vi "Acquire Data.vi"(7 "Total Buffer Size":i32, 8 "error in (no error)":errorcluster, 10 "Acquisition and Logging Configuration":T1={"Data Rate"=1, "Samples per Read"=0, "Number of Reads to Save"=0, "Data File Name"="", "TDMS Properties"=[], "Number of Channels"=4, "Channel Scale Array"=[0.0, 0.0, 0.0, 0.0], "Channel Names"=[], "Trigger - RMS Value"=0.0, "Trigger - Channel"=0, "Trigger - Time (Minute)"=0} {"Data Rate" items=["51.200 kS/s (NI 9234)"=1, "25.600 kS/s (NI 9234)"=2, "17.067 kS/s (NI 9234)"=3, "12.800 kS/s (NI 9234)"=4, "10.240 kS/s (NI 9234)"=5, "8.533 kS/s (NI 9234)"=6, "7.314 kS/s (NI 9234)"=7, "6.400 kS/s (NI 9234)"=8, "5.689 kS/s (NI 9234)"=9, "5.120 kS/s (NI 9234)"=10, "4.654 kS/s (NI 9234)"=11, "4.267 kS/s (NI 9234)"=12, "3.938 kS/s (NI 9234)"=13, "3.657 kS/s (NI 9234)"=14, "3.413 kS/s (NI 9234)"=15, "3.200 kS/s (NI 9234)"=16, "3.012 kS/s (NI 9234)"=17, "2.845 kS/s (NI 9234)"=18, "2.695 kS/s (NI 9234)"=19, "2.560 kS/s (NI 9234)"=20, "2.438 kS/s (NI 9234)"=21, "2.328 kS/s (NI 9234)"=22, "2.226 kS/s (NI 9234)"=23, "2.133 kS/s (NI 9234)"=24, "2.048 kS/s (NI 9234)"=25, "1.969 kS/s (NI 9234)"=26, "1.896 kS/s (NI 9234)"=27, "1.829 kS/s (NI 9234)"=28, "1.765 kS/s (NI 9234)"=29, "1.707 kS/s (NI 9234)"=30, "1.652 kS/s (NI 9234)"=31]}, 11 "FPGA VI Reference":T4) -> (0 "error out":errorcluster, 1 "Waveform Data":waveform(sgl)[](array[waveform]), 2 "dup Acquisition and Logging Configuration":T1={"Data Rate"=1, "Samples per Read"=0, "Number of Reads to Save"=0, "Data File Name"="", "TDMS Properties"=[], "Number of Channels"=4, "Channel Scale Array"=[0.0, 0.0, 0.0, 0.0], "Channel Names"=[], "Trigger - RMS Value"=0.0, "Trigger - Channel"=0, "Trigger - Time (Minute)"=0} {"Data Rate" items=["51.200 kS/s (NI 9234)"=1, "25.600 kS/s (NI 9234)"=2, "17.067 kS/s (NI 9234)"=3, "12.800 kS/s (NI 9234)"=4, "10.240 kS/s (NI 9234)"=5, "8.533 kS/s (NI 9234)"=6, "7.314 kS/s (NI 9234)"=7, "6.400 kS/s (NI 9234)"=8, "5.689 kS/s (NI 9234)"=9, "5.120 kS/s (NI 9234)"=10, "4.654 kS/s (NI 9234)"=11, "4.267 kS/s (NI 9234)"=12, "3.938 kS/s (NI 9234)"=13, "3.657 kS/s (NI 9234)"=14, "3.413 kS/s (NI 9234)"=15, "3.200 kS/s (NI 9234)"=16, "3.012 kS/s (NI 9234)"=17, "2.845 kS/s (NI 9234)"=18, "2.695 kS/s (NI 9234)"=19, "2.560 kS/s (NI 9234)"=20, "2.438 kS/s (NI 9234)"=21, "2.328 kS/s (NI 9234)"=22, "2.226 kS/s (NI 9234)"=23, "2.133 kS/s (NI 9234)"=24, "2.048 kS/s (NI 9234)"=25, "1.969 kS/s (NI 9234)"=26, "1.896 kS/s (NI 9234)"=27, "1.829 kS/s (NI 9234)"=28, "1.765 kS/s (NI 9234)"=29, "1.707 kS/s (NI 9234)"=30, "1.652 kS/s (NI 9234)"=31]})   [LabVIEW 2012]
doc: "Reads waveform data from the DMA FIFO."
uses:
  LabVIEW Data/FPGA Logging Test/controls/FPGA VI Reference.ctl
  LabVIEW Data/FPGA Logging Test/controls/Acquisition and Logging Configuration.ctl
  <vilib>/LabVIEW Targets/FPGA/cRIO/shared/nicrio_ModuleControls/nicrio_cRIO-9234_DataRatesRing2.ctl
  LabVIEW Data/FPGA Logging Test/controls/TDMS Properties.ctl
  LabVIEW Data/FPGA Logging Test/Globals/Global - Monitoring Variables.vi
  <vilib>/Utility/error.llb/Error Cluster From Error Code.vi
  <vilib>/rvi/errors/niLvFpgaAdjustHostInterfaceError.vi
  <vilib>/rvi/interface/nirviReadWriteControl/nirviReadWriteControl.xnode
  <vilib>/rvi/interface/nirviMethod/nirviMethod.xnode
  NiFpgaLv.dll
  <vilib>/rvi/interface/Simulation/niFpgaSimulationCallBeginRW.vi
  <vilib>/FPGAPlugInAG/Dynamic/niLvFpga_ReadFifo_Dynamic.vi
  <vilib>/rvi/errors/niLvFpgaMergeErrorWithErrorCode.vi
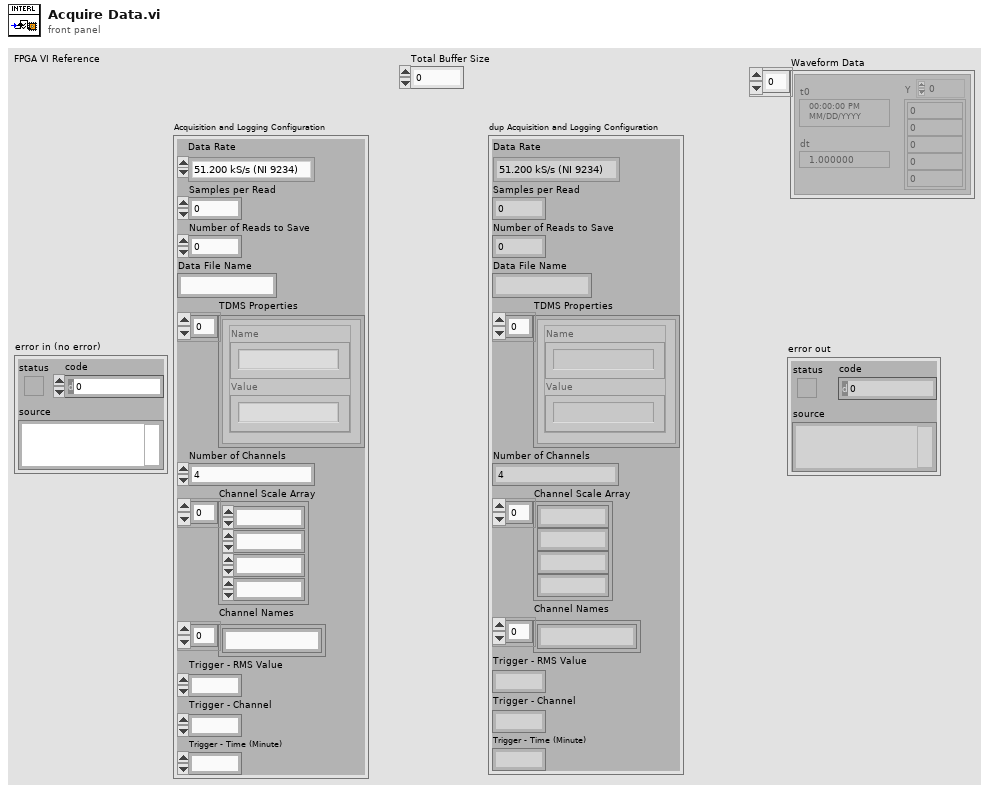
[diagram p1: front panel]
types:
  T1 = typedef "Acquisition and Logging Configuration.ctl" = cluster{"Data Rate":T2, "Samples per Read":i32, "Number of Reads to Save":i32, "Data File Name":string, "TDMS Properties":T3[], "Number of Channels":i32, "Channel Scale Array":fxp<+,24,12>[], "Channel Names":string[], "Trigger - RMS Value":dbl, "Trigger - Channel":i32, "Trigger - Time (Minute)":i32}
  T2 = typedef "nicrio_cRIO-9234_DataRatesRing2.ctl" = u8
  T3 = typedef "TDMS Properties.ctl" = cluster{"Name":string, "Value":string}
  T4 = typedef "FPGA VI Reference.ctl" = refnum<k20>
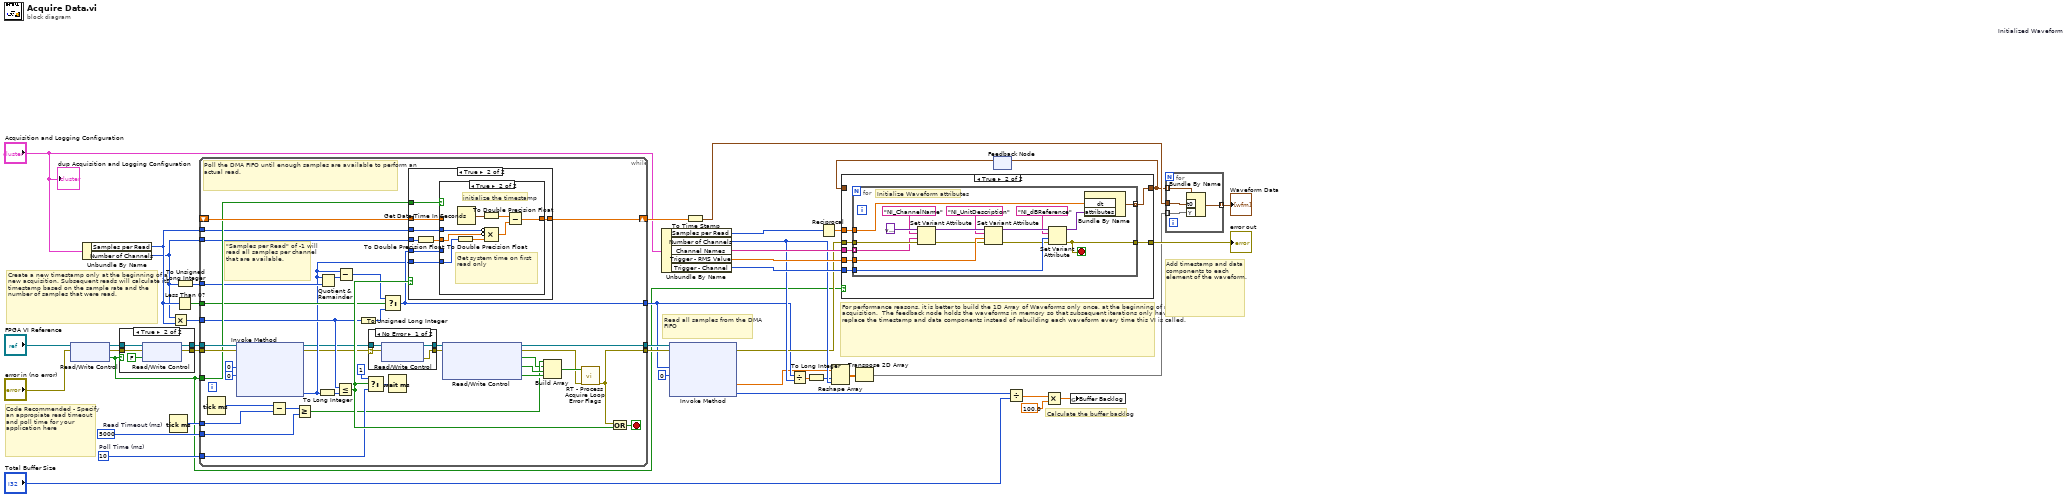
[diagram p0: block diagram]
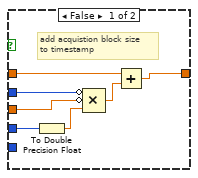
[diagram p5: hidden frame]
diagram:
  w13 = u32 10  # Poll Time (ms)
  w14 = u32 5000  # Read Timeout (ms)
  # "Calculate the buffer backlog"
  # "For performance reasons, it is better to build the 1D Array of Waveforms only once, at the beginning of an acquisition.  The feedback node holds the waveforms in memory so that subsequent iterations only have to replace the timestamp and data components instead of rebuilding each waveform every time this VI is called."
  # "Read all samples from the DMA FIFO"
  # "Code Recommended - Specify an appropiate read timeout and poll time for your application here"
  # "Create a new timestamp only at the beginning of a new acquisition. Subsequent reads will calculate its timestamp based on the sample rate and the number of samples that were read."
  # "Add timestamp and data components to each element of the waveform."
  n1 = xnode "Read/Write Control"("FPGA VI Reference In"="FPGA VI Reference", "error in"="error in (no error)") -> ("FPGA VI Reference Out"=w42:T4, "error out"=w43:errorcluster, "First Read"=w8:bool)
  n2 = Unbundle By Name("Acquisition and Logging Configuration") -> ("Samples per Read"=w16:i32, "Number of Channels"=w15:i32)
  n3 = case shown="True" w8 {
    tunnel: w42 -> [w45 w50]
    tunnel: [w45 w49] -> w40
    tunnel: w43 -> [w44 w48]
    tunnel: [w44 w47] -> w39
    frame False {
    }
    frame True {
      n4 = xnode "Read/Write Control"("FPGA VI Reference In"=w50, "error in"=w48, "First Read"=FALSE) -> ("FPGA VI Reference Out"=w49:T4, "error out"=w47:errorcluster)
    }
  }
  n5 = Tick Count (ms)() -> (millisecond timer value=w38:u32)
  n6 = Multiply(x=w15, y=w16) -> (x*y=w27:i32)
  n7 = Less Than 0?(x=w16) -> (x < 0?=w28:bool)
  n8 = To Unsigned Long Integer(number=w15) -> (unsigned 32bit integer=w26:u32)
  n9 = while {
    tunnel: [w52] -> w34
    tunnel: [w58] -> w35
    tunnel: w8 -> [w84]
    tunnel: w40 -> [w87]
    tunnel: w39 -> [w86]
    shift-right: [w79] -> w32
    shift-left: _ -> [w85]
    tunnel: w38 -> [w88]
    tunnel: w27 -> [w75]
    tunnel: [w73] -> w12
    tunnel: w28 -> [w78]
    tunnel: w26 -> [w74]
    tunnel: w16 -> [w66]
    tunnel: w15 -> [w65]
    tunnel: w14 -> [w64]
    tunnel: w13 -> [w63]
    stop <- w89 stop-if-true
    # "\"Samples per Read\" of -1 will read all samples per channel that are available."
    # "Poll the DMA FIFO until enough samples are available to perform an actual read."
    n10 = Tick Count (ms)() -> (millisecond timer value=w83:u32)
    n11 = xnode "Invoke Method"("FPGA VI Reference In"=w87, "error in"=w86, "Number of Elements"=u32 0, "Timeout (ms)"=0) -> ("FPGA VI Reference Out"=w61:T4, "error out"=w62:errorcluster, "Elements Remaining"=w68:u32)  [unwired: 1 out]
    n12 = Subtract(x=w83, y=w88) -> (x-y=w67:u32)
    n13 = Greater Or Equal?(x=w67, y=w64) -> (x >= y?=w55:bool)
    n14 = To Long Integer(number=w68) -> (32bit integer=w77:i32)
    n15 = Quotient & Remainder(x=w68, y=w74) -> (x-y*floor(x/y)=w72:u32)  [unwired: 1 out]
    n16 = Less Or Equal?(x=w75, y=w77) -> (x <= y?=w82:bool)
    n17 = Subtract(x=w68, y=w72) -> (x-y=w71:u32)
    n18 = To Unsigned Long Integer(number=w75) -> (unsigned 32bit integer=w76:u32)
    n19 = Select(t=u32 1, s=w82, f=w63) -> (s? t:f=w81:u32)
    n20 = case shown="No Error" w62 {
      selector: w62 -> [w93 w94]
      tunnel: w61 -> [w92 w95]
      tunnel: [w91 w95] -> w60
      tunnel: [w90 w94] -> w59
      frame No Error {
        n21 = xnode "Read/Write Control"("FPGA VI Reference In"=w92, "error in"=w93) -> ("FPGA VI Reference Out"=w91:T4, "FPGA Error"=w90:errorcluster)  [unwired: 1 out]
      }
      frame Error {
      }
    }
    n22 = Select(t=w71, s=w78, f=w76) -> (s? t:f=w73:u32)
    n23 = Wait (ms)(milliseconds to wait=w81) -> ()  [unwired: 1 out]
    n24 = case shown="True" w82 {
      tunnel: w85 -> [w96 w104]
      tunnel: w84 -> [_ w103]
      tunnel: w68 -> [_ w102]
      tunnel: [w96 w101] -> w79
      tunnel: w73 -> [_ w100]
      tunnel: w66 -> [_ w98]
      tunnel: w65 -> [_ w97]
      frame False {
      }
      frame True {
        n25 = To Double Precision Float(number=w97) -> (double precision float=w99:dbl)
        n26 = case shown="True" w103 {
          tunnel: w98 -> [w109 w119]
          tunnel: w104 -> [w110 _]
          tunnel: w100 -> [w106 _]
          tunnel: w99 -> [w107 w118]
          tunnel: w102 -> [_ w113]
          tunnel: [w111 w115] -> w101
          frame False {
            # "add acquistion block size\nto timestamp"
            n27 = To Double Precision Float(number=w106) -> (double precision float=w105:dbl)
            n28 = Compound Arithmetic op=MULTIPLY(invert w109, invert w107, w105) -> (w108:dbl)
            n29 = Add(x=w110, y=w108) -> (x+y=w111:dbl)
          }
          frame True {
            # "Get system time on first read only"
            # "initialize the timestamp"
            n30 = To Double Precision Float(number=w113) -> (double precision float=w112:dbl)
            n31 = Get Date/Time In Seconds() -> (seconds since 1Jan1904=w117:timestamp)
            n32 = To Double Precision Float(number=w117) -> (double precision float=w114:dbl)
            n33 = Compound Arithmetic op=MULTIPLY(invert w119, invert w118, w112) -> (w116:dbl)
            n34 = Subtract(x=w114, y=w116) -> (x-y=w115:dbl)
          }
        }
      }
    }
    n35 = xnode "Read/Write Control"("FPGA VI Reference In"=w60, "error in"=w59) -> ("FPGA VI Reference Out"=w58:T4, "error out"=w51:errorcluster, "Module Underflow"=w54:bool, "DMA FIFO Full"=w57:bool, "Different Channel Count"=w56:bool)
    n36 = Build Array(w55, w54, w57, w56) -> (w53:bool[])
    n37 = call "RT - Process Acquire Loop Error Flags.vi"("error in (no error)"=w51, "Error Flags"=w53) -> ("error out"=w52:errorcluster)  [unwired: 9 in]
    n38 = Compound Arithmetic op=OR(w52, w82) -> (w89:bool)
  }
  n39 = Unbundle By Name("Acquisition and Logging Configuration") -> ("Samples per Read"=w37:i32, "Number of Channels"=w25:i32, "Channel Names"=w29:string[], "Trigger - RMS Value"=w30:dbl, "Trigger - Channel"=w33:i32)
  n40 = xnode "Invoke Method"("FPGA VI Reference In"=w35, "error in"=w34, "Number of Elements"=w12, "Timeout (ms)"=0) -> ("error out"=w18:errorcluster, "Data"=w1:sgl[], "Elements Remaining"=w6:u32)  [unwired: 1 out]
  n41 = To Time Stamp(1:w32) -> (0:w11:timestamp)
  n42 = Divide(x=w12, y=w25) -> (x/y=w24:dbl)
  n43 = To Long Integer(number=w24) -> (32bit integer=w23:i32)
  n44 = Reciprocal(x=w37) -> (1/x=w36:dbl)
  n45 = Reshape Array(w1, w23, w25) -> (w21:sgl[][])
  n46 = Transpose 2D Array(2D array=w21) -> (transposed array=w20:sgl[][])
  n47 = feedback #1 "Initialized Waveforms"() -> (w9:waveform(sgl)[])  [unwired: 1 in]
  n48 = case shown="True" w8 {
    tunnel: w36 -> [_ w128]
    tunnel: w33 -> [_ w127]
    tunnel: w18 -> [w121 w126]
    tunnel: [w121 w125] -> w31
    tunnel: w30 -> [_ w124]
    tunnel: w29 -> [_ w123]
    tunnel: [w120 w122] -> w10
    tunnel: w9 -> [w120 _]
    frame False {
    }
    frame True {
      n49 = for {
        tunnel: w128 -> [w144]
        tunnel: [w143] -> w122 mode=indexing
        tunnel: w124 -> [w141]
        tunnel: w127 -> [w139]
        tunnel: w126 -> [w140]
        tunnel: [w129] -> w125
        tunnel: w123 -> [w130] mode=indexing
        stop <- w129 stop-if-true
        # "Initialize Waveform attributes"
        n50 = Set Variant Attribute(Variant=variant ("variant out"), name="NI_ChannelName", value=w130, error in=w140) -> (Variant out=w135:variant, error out=w137:errorcluster)  [unwired: 1 out]
        n51 = Set Variant Attribute(Variant=w135, name="NI_UnitDescription", value=w141, error in=w137) -> (Variant out=w136:variant, error out=w138:errorcluster)  [unwired: 1 out]
        n52 = Set Variant Attribute(Variant=w136, name="NI_dBReference", value=w139, error in=w138) -> (Variant out=w142:variant, error out=w129:errorcluster)  [unwired: 1 out]
        n53 = Bundle By Name("dt"=w144, "attributes"=w142) -> (w143:waveform(sgl))  [unwired: 1 out]
      }
    }
  }
  "error out" <- w31
  n54 = feedback-in #1(w10) -> ()
  n55 = Divide(x=w6, y="Total Buffer Size") -> (x/y=w7:dbl)
  n56 = Multiply(x=w7, y=100.0) -> (x*y=w4:dbl)
  n57 = global write "Global - Monitoring Variables.vi" "Buffer Backlog"(w4) -> ()
  n58 = for {
    tunnel: w10 -> [w148] mode=indexing
    tunnel: w11 -> [w147]
    tunnel: [w146] -> w22 mode=indexing
    tunnel: w20 -> [w145] mode=indexing
    n59 = Bundle By Name(cluster=w148, "t0"=w147, "Y"=w145) -> (w146:waveform(sgl))
  }
  "Waveform Data" <- w22
  "dup Acquisition and Logging Configuration" <- "Acquisition and Logging Configuration"
